vi "Diagonal Vents.vi"() -> ()   [LabVIEW 2020]
uses:
  <vilib>/regexp/Match Regular Expression.xnode
panel:
  out "Array":i32[][](array[numeric])
  out "Count":i32
  in  "Input":string="599,531 -> 599,32\n435,904 -> 435,489\n768,714 -> 768,187\n845,552 -> 596,801\n167,680 -> 167,445\n45,887 -> 45,346\n780,295 -> 179,896\n310,539 -> 602,831\n535,556 -> 349,556\n797,180 -> 797,62\n771,406 -> 120,406\n383,296 -> 383,918\n689,815 -> 73,199\n658,642 -> 658,333\n931,104 -> 708,104\n406,278 -> 406,29\n315,532 -> 773,74\n439,953 -> 289,953\n555,162 -> 695,302\n444,522 -> 444,828\n460,844 -> 460,972\n838,18 -> 143,713\n335,785 -> 335,485\n757,886 -> 757,327\n266,205 -> 273,205\n934,42 -> 19,957\n671,622 -> 263,214\n739,781 -> 739,332\n848,507 -> 848,394\n577,58 -> 461,174\n49,905 -> 921,33\n627,455 -> 205,455\n106,523 -> 974,523\n707,335 -> 707,313\n65,214 -> 712,214\n610,267 -> 610,403\n47,699 -> 565,181\n288,833 -> 709,833\n452,59 -> 452,632\n629,209 -> 125,209\n535,232 -> 535,342\n542,942 -> 542,753\n618,905 -> 552,905\n598,314 -> 976,314\n350,824 -> 17,824\n753,570 -> 753,617\n544,302 -> 259,302\n628,271 -> 628,379\n856,265 -> 856,792\n77,317 -> 77,122\n905,420 -> 905,687\n812,512 -> 812,411\n844,486 -> 771,559\n798,778 -> 798,215\n571,160 -> 278,453\n242,352 -> 227,352\n958,118 -> 167,909\n201,915 -> 201,564\n163,583 -> 163,279\n23,111 -> 23,883\n248,281 -> 331,281\n381,768 -> 900,768\n78,988 -> 78,326\n914,659 -> 247,659\n532,531 -> 520,531\n65,309 -> 734,978\n170,923 -> 399,694\n740,496 -> 196,496\n832,452 -> 816,452\n675,463 -> 878,463\n659,852 -> 560,852\n143,655 -> 227,655\n334,795 -> 334,978\n217,913 -> 368,913\n675,33 -> 503,33\n42,981 -> 811,981\n458,162 -> 722,162\n92,613 -> 92,542\n393,584 -> 393,252\n276,256 -> 725,705\n752,442 -> 752,789\n63,281 -> 744,281\n596,845 -> 35,284\n594,534 -> 964,164\n337,380 -> 337,511\n158,142 -> 75,225\n606,47 -> 606,111\n987,30 -> 62,955\n192,196 -> 428,196\n449,672 -> 449,77\n804,151 -> 804,255\n783,581 -> 287,581\n860,891 -> 69,100\n966,187 -> 761,392\n400,742 -> 278,742\n661,656 -> 592,587\n787,415 -> 787,771\n866,228 -> 417,228\n915,385 -> 505,385\n715,620 -> 715,633\n615,31 -> 615,940\n691,885 -> 527,885\n426,705 -> 351,705\n258,215 -> 258,949\n480,449 -> 480,710\n788,710 -> 788,67\n850,90 -> 597,90\n398,379 -> 18,759\n248,107 -> 665,524\n901,933 -> 208,240\n433,424 -> 110,424\n214,447 -> 389,272\n468,330 -> 468,928\n950,759 -> 332,759\n447,541 -> 420,541\n659,138 -> 604,83\n821,264 -> 95,264\n914,132 -> 46,132\n821,604 -> 821,57\n805,734 -> 85,14\n806,274 -> 164,916\n205,780 -> 205,133\n798,472 -> 361,472\n817,57 -> 127,747\n172,119 -> 922,869\n118,167 -> 55,167\n56,548 -> 344,836\n117,108 -> 940,931\n530,46 -> 530,785\n528,507 -> 729,708\n11,986 -> 987,10\n979,932 -> 76,29\n863,250 -> 210,903\n879,215 -> 891,215\n592,219 -> 592,528\n211,760 -> 211,347\n21,842 -> 633,230\n110,356 -> 110,254\n925,606 -> 444,125\n757,566 -> 757,498\n702,622 -> 637,622\n51,379 -> 365,379\n273,906 -> 273,494\n170,795 -> 929,36\n159,56 -> 435,56\n724,953 -> 724,735\n536,748 -> 901,748\n937,148 -> 937,510\n963,507 -> 863,507\n840,290 -> 840,221\n864,154 -> 55,963\n977,487 -> 685,487\n863,617 -> 210,617\n862,308 -> 291,879\n286,477 -> 286,276\n550,805 -> 550,489\n964,508 -> 821,651\n475,290 -> 789,290\n25,882 -> 25,349\n570,374 -> 604,374\n354,442 -> 514,282\n457,700 -> 360,700\n548,889 -> 548,502\n11,393 -> 11,829\n60,714 -> 781,714\n943,953 -> 972,924\n757,386 -> 465,386\n230,463 -> 27,463\n815,385 -> 326,385\n32,630 -> 378,976\n298,853 -> 298,644\n532,146 -> 23,146\n958,685 -> 737,464\n853,847 -> 79,73\n815,590 -> 815,961\n49,87 -> 751,789\n55,513 -> 55,378\n163,907 -> 574,907\n355,168 -> 355,836\n453,742 -> 674,742\n273,458 -> 685,458\n981,961 -> 958,984\n120,59 -> 401,59\n735,964 -> 395,964\n277,377 -> 277,646\n633,694 -> 633,707\n224,376 -> 976,376\n201,790 -> 293,790\n950,952 -> 12,14\n389,48 -> 356,48\n337,424 -> 166,424\n591,915 -> 591,456\n205,162 -> 942,162\n404,421 -> 404,748\n319,983 -> 608,694\n94,677 -> 94,853\n873,388 -> 873,617\n858,82 -> 858,890\n64,503 -> 64,787\n372,224 -> 50,546\n531,241 -> 960,670\n47,33 -> 975,961\n853,52 -> 271,634\n668,437 -> 668,719\n162,290 -> 843,290\n421,299 -> 944,822\n103,983 -> 103,324\n290,71 -> 290,686\n209,38 -> 546,38\n740,878 -> 378,878\n741,795 -> 741,916\n27,431 -> 445,431\n795,289 -> 795,759\n345,772 -> 775,772\n977,480 -> 512,15\n49,863 -> 49,659\n223,590 -> 779,590\n503,771 -> 917,771\n499,289 -> 935,725\n246,459 -> 246,395\n860,257 -> 656,257\n425,87 -> 425,603\n355,378 -> 355,23\n462,286 -> 462,358\n181,571 -> 181,732\n17,649 -> 476,649\n394,321 -> 394,293\n812,660 -> 515,957\n21,150 -> 799,928\n437,593 -> 437,372\n125,495 -> 373,743\n482,404 -> 482,420\n283,580 -> 283,234\n667,966 -> 827,806\n959,961 -> 959,931\n461,845 -> 206,845\n299,888 -> 299,836\n680,828 -> 680,855\n958,977 -> 26,45\n847,419 -> 290,976\n892,920 -> 892,180\n487,945 -> 487,445\n329,570 -> 583,570\n110,940 -> 989,61\n475,351 -> 882,351\n953,229 -> 429,229\n119,125 -> 749,125\n834,103 -> 212,725\n978,412 -> 978,343\n916,310 -> 758,310\n825,761 -> 720,761\n353,954 -> 353,795\n422,464 -> 422,356\n662,964 -> 836,790\n242,873 -> 242,570\n742,972 -> 797,972\n698,364 -> 360,26\n258,633 -> 19,872\n406,649 -> 406,685\n386,710 -> 925,710\n347,657 -> 524,480\n812,905 -> 554,647\n420,505 -> 420,231\n908,693 -> 908,724\n130,772 -> 130,898\n560,23 -> 560,987\n941,831 -> 941,544\n817,940 -> 132,255\n515,280 -> 515,811\n544,102 -> 568,102\n115,612 -> 67,660\n743,762 -> 743,152\n246,14 -> 691,459\n766,492 -> 673,492\n467,179 -> 351,63\n655,779 -> 655,524\n314,171 -> 314,108\n414,64 -> 502,64\n564,239 -> 894,239\n984,974 -> 56,46\n201,963 -> 201,223\n238,194 -> 238,832\n30,652 -> 477,652\n818,735 -> 582,971\n225,566 -> 673,566\n172,865 -> 74,865\n264,101 -> 264,812\n487,916 -> 979,916\n879,30 -> 10,899\n797,657 -> 797,136\n750,642 -> 593,799\n550,244 -> 418,376\n158,816 -> 668,816\n505,648 -> 303,648\n411,688 -> 263,688\n544,35 -> 771,35\n545,846 -> 286,846\n284,760 -> 284,929\n835,401 -> 708,401\n533,591 -> 545,591\n866,757 -> 475,757\n202,62 -> 907,767\n456,655 -> 456,123\n367,714 -> 225,714\n359,679 -> 926,679\n623,853 -> 623,865\n170,120 -> 213,120\n481,741 -> 481,435\n928,73 -> 41,960\n551,282 -> 551,265\n988,986 -> 12,10\n351,172 -> 791,172\n49,65 -> 952,968\n725,617 -> 691,617\n509,159 -> 697,159\n83,985 -> 83,968\n206,617 -> 334,489\n880,682 -> 966,768\n60,896 -> 60,617\n501,686 -> 49,234\n801,708 -> 738,771\n548,883 -> 548,33\n753,162 -> 29,162\n102,478 -> 102,295\n115,656 -> 637,134\n924,970 -> 924,963\n191,340 -> 191,515\n764,481 -> 523,481\n97,619 -> 97,890\n228,183 -> 228,624\n171,867 -> 68,867\n797,685 -> 167,685\n510,955 -> 464,955\n930,955 -> 233,258\n934,572 -> 934,900\n217,822 -> 797,242\n868,939 -> 369,440\n861,811 -> 861,36\n346,617 -> 346,153\n754,526 -> 754,426\n482,724 -> 482,21\n328,984 -> 976,984\n933,895 -> 325,287\n965,973 -> 232,240\n502,707 -> 767,972\n353,680 -> 815,218\n311,210 -> 311,157\n156,944 -> 928,172\n615,395 -> 101,909\n107,500 -> 528,921\n375,42 -> 375,796\n13,292 -> 818,292\n613,144 -> 613,541\n340,677 -> 340,406\n631,655 -> 744,655\n22,242 -> 723,943\n705,596 -> 980,321\n316,955 -> 316,515\n760,279 -> 44,279\n391,328 -> 391,724\n917,476 -> 917,668\n66,907 -> 913,60\n597,260 -> 362,25\n568,584 -> 568,297\n375,506 -> 375,300\n988,31 -> 72,947\n425,342 -> 154,342\n196,395 -> 899,395\n904,17 -> 94,17\n546,159 -> 751,159\n284,557 -> 175,448\n69,201 -> 697,201\n130,421 -> 224,421\n646,462 -> 637,453\n187,638 -> 621,638\n832,212 -> 416,212\n614,582 -> 348,582\n677,404 -> 677,709\n178,122 -> 915,859\n81,849 -> 223,849\n717,18 -> 646,18\n723,666 -> 974,666\n703,234 -> 130,234\n317,107 -> 106,107\n207,397 -> 207,375\n688,465 -> 982,171\n749,201 -> 610,201\n280,313 -> 827,860\n773,873 -> 917,873\n337,908 -> 337,155\n541,427 -> 385,583\n611,314 -> 131,794\n966,909 -> 104,47\n785,556 -> 346,556\n914,645 -> 914,718\n683,941 -> 657,915\n919,665 -> 310,56\n743,978 -> 779,978\n953,925 -> 953,854\n899,347 -> 705,347\n46,597 -> 46,255\n332,364 -> 922,954\n38,987 -> 832,193\n77,585 -> 77,262\n155,61 -> 734,640\n953,136 -> 655,136\n939,730 -> 158,730\n903,458 -> 393,458\n50,227 -> 50,249\n536,814 -> 536,242\n906,694 -> 259,47\n317,237 -> 853,773\n828,55 -> 509,55\n40,664 -> 341,965\n414,820 -> 53,459\n244,344 -> 272,344\n191,606 -> 308,606\n329,409 -> 329,960\n166,863 -> 938,91\n655,396 -> 291,760\n634,666 -> 625,666\n360,622 -> 360,550\n568,473 -> 840,201\n534,162 -> 534,823\n583,563 -> 583,521\n124,447 -> 124,79\n207,559 -> 207,649\n688,238 -> 26,900\n173,33 -> 117,33\n665,800 -> 665,86\n121,515 -> 121,132\n32,472 -> 32,960\n513,28 -> 513,299\n881,612 -> 881,415\n72,71 -> 977,976\n169,821 -> 111,821\n603,756 -> 254,756\n182,129 -> 182,824\n746,670 -> 942,670\n143,15 -> 72,86\n108,134 -> 963,989\n860,388 -> 834,362\n252,811 -> 473,811\n575,306 -> 575,368\n686,471 -> 686,38\n673,59 -> 673,861\n461,949 -> 491,949\n915,373 -> 330,958\n933,699 -> 588,699\n254,798 -> 254,498\n329,865 -> 329,926\n569,243 -> 659,243\n762,808 -> 921,967\n722,460 -> 68,460\n136,470 -> 355,470\n133,919 -> 56,842\n87,868 -> 853,102\n622,102 -> 446,102\n798,494 -> 135,494\n281,858 -> 281,172\n141,172 -> 765,796\n794,194 -> 102,886\n539,983 -> 539,895\n841,755 -> 841,365\n695,429 -> 166,958\n965,933 -> 899,933\n603,699 -> 603,708\n598,635 -> 844,635\n288,190 -> 288,946\n559,383 -> 423,383\n795,332 -> 409,718\n600,645 -> 478,645\n831,24 -> 905,24\n13,817 -> 606,224\n828,878 -> 96,146\n32,197 -> 32,891\n84,832 -> 84,756\n404,281 -> 404,781\n394,441 -> 489,536\n845,876 -> 589,876\n833,114 -> 833,834\n979,130 -> 979,238\n907,189 -> 396,700\n448,740 -> 714,474\n145,837 -> 100,837\n982,983 -> 38,39\n962,506 -> 962,764\n773,922 -> 975,922\n892,666 -> 904,654\n754,201 -> 459,496\n108,829 -> 108,894\n122,381 -> 122,484\n683,301 -> 630,354\n47,103 -> 897,953\n549,880 -> 942,487\n944,15 -> 44,915\n713,456 -> 713,402\n83,865 -> 239,865\n814,585 -> 814,105\n980,439 -> 685,439"
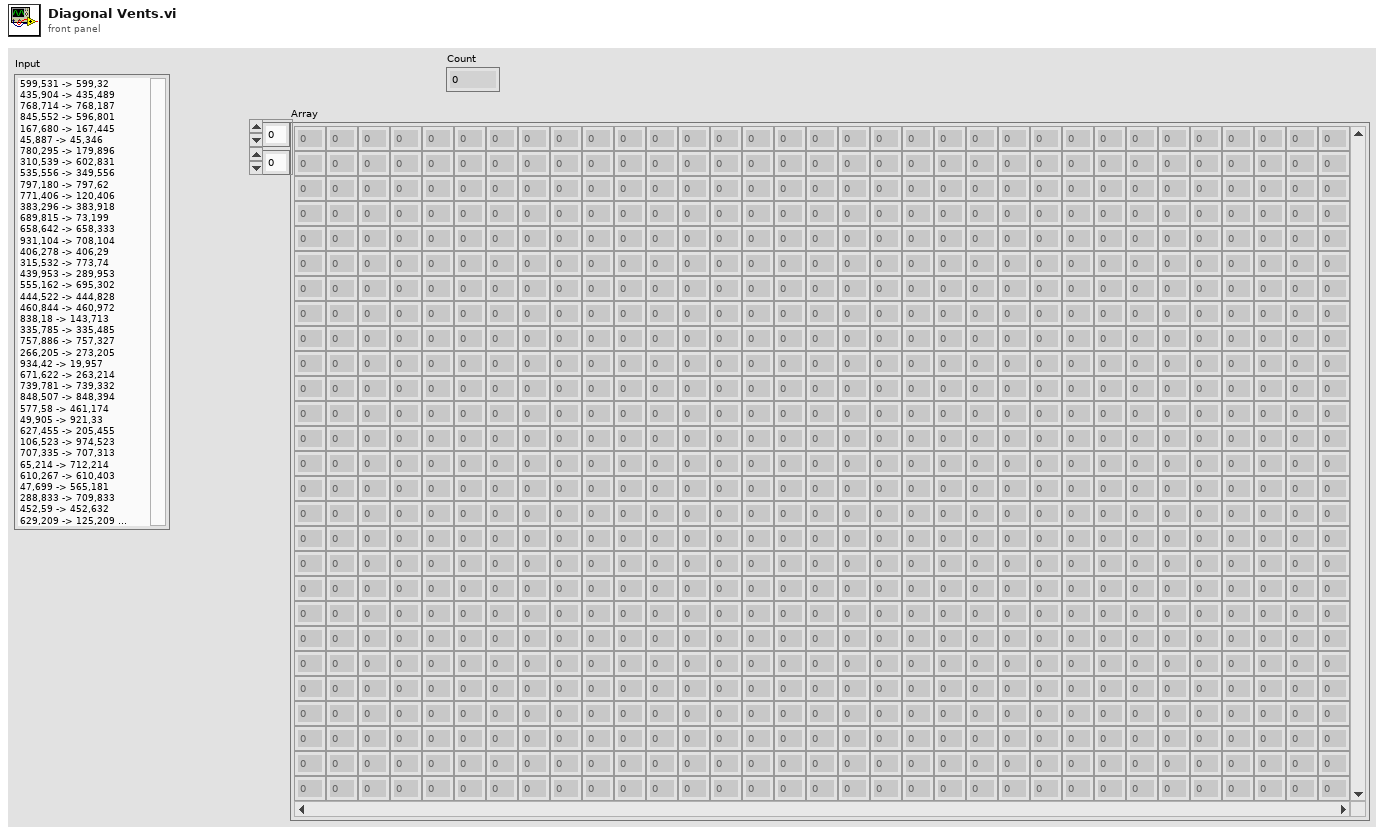
[diagram p1: front panel]
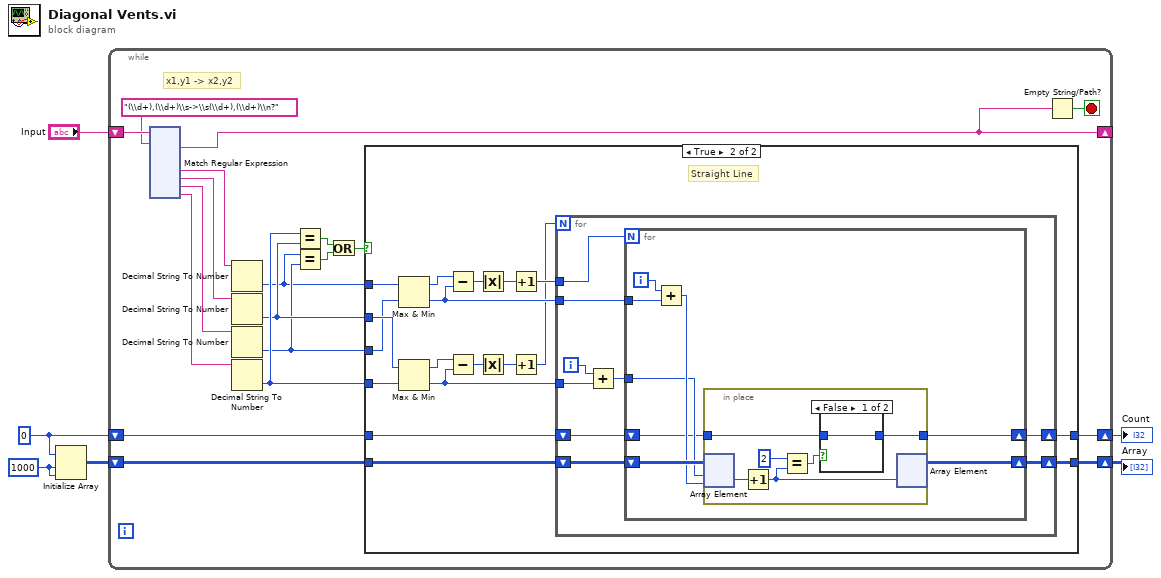
[diagram p0: block diagram]
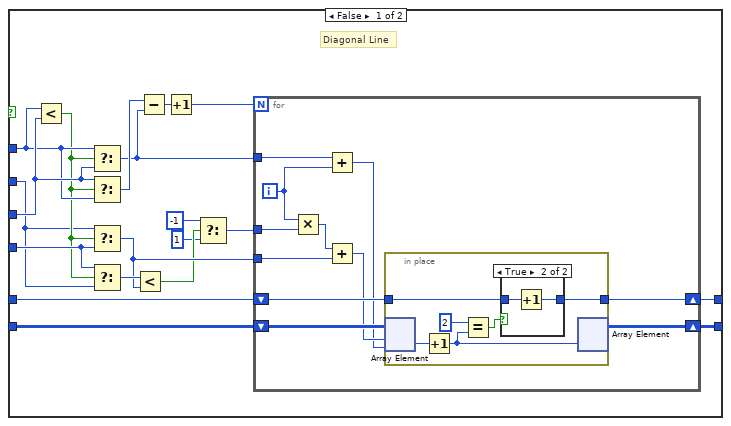
[diagram p2: hidden frame]
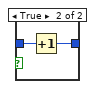
[diagram p4: hidden frame]
diagram:
  w3 = 0
  w6 = 1000 ("dimension size")
  n1 = Initialize Array(w3, w6, w6) -> (w4:i32[][])
  n2 = while {
    shift-right: [w19] -> _
    shift-left: "Input" -> [w25]
    shift-right: [w15] -> w1
    shift-left: w4 -> [w16]
    shift-right: [w14] -> w2
    shift-left: w3 -> [w17]
    stop <- w18 stop-if-true
    # "x1,y1 -> x2,y2"
    n3 = xnode "Match Regular Expression"("input string"=w25, "regular expression"="(\\d+),(\\d+)\\s->\\s(\\d+),(\\d+)\\n?") -> ("after match"=w19:string, "submatch 1"=w23:string, "submatch 2"=w22:string, "submatch 3"=w21:string, "submatch 4"=w20:string)  [unwired: 4 in, 4 out]
    n4 = Decimal String To Number(string=w23) -> (number=w7:i32)  [unwired: 2 in, 1 out]
    n5 = Decimal String To Number(string=w22) -> (number=w9:i32)  [unwired: 2 in, 1 out]
    n6 = Decimal String To Number(string=w21) -> (number=w8:i32)  [unwired: 2 in, 1 out]
    n7 = Decimal String To Number(string=w20) -> (number=w10:i32)  [unwired: 2 in, 1 out]
    n8 = Equal?(x=w10, y=w9) -> (x = y?=w13:bool)
    n9 = Equal?(x=w7, y=w8) -> (x = y?=w12:bool)
    n10 = Or(x=w13, y=w12) -> (x .or. y?=w11:bool)
    n11 = case shown="True" w11 {
      tunnel: w17 -> [w163 w201]
      tunnel: w16 -> [w162 w200]
      tunnel: [w160 w199] -> w15
      tunnel: [w161 w198] -> w14
      tunnel: w10 -> [w153 w191]
      tunnel: w9 -> [w151 w190]
      tunnel: w8 -> [w159 w189]
      tunnel: w7 -> [w158 w188]
      frame False {
        # "Diagonal Line"
        n12 = Less?(x=w158, y=w159) -> (x < y?=w152:bool)
        n13 = Select(t=w158, s=w152, f=w159) -> (s? t:f=w154:i32)
        n14 = Select(t=w159, s=w152, f=w158) -> (s? t:f=w157:i32)
        n15 = Select(t=w151, s=w152, f=w153) -> (s? t:f=w148:i32)
        n16 = Select(t=w153, s=w152, f=w151) -> (s? t:f=w150:i32)
        n17 = Less?(x=w150, y=w148) -> (x < y?=w147:bool)
        n18 = Subtract(x=w157, y=w154) -> (x-y=w156:i32)
        n19 = Increment(x=w156) -> (x+1=w155:i32)
        n20 = Select(t=-1, s=w147, f=1) -> (s? t:f=w149:i32)
        n21 = for {
          N: w155 -> [_]
          tunnel: w154 -> [w174]
          tunnel: w148 -> [w173]
          shift-right: [w168] -> w161
          shift-left: w163 -> [w171]
          shift-right: [w164] -> w160
          shift-left: w162 -> [w172]
          tunnel: w149 -> [w165]
          i -> [w166]
          n22 = Multiply(x=w166, y=w165) -> (x*y=w167:i32)
          n23 = Add(x=w174, y=w166) -> (x+y=w169:i32)
          n24 = Add(x=w167, y=w173) -> (x+y=w170:i32)
          n25 = in-place {
            in-place-border: w171 -> [w176]
            in-place-border: [w175] -> w168
            n26 = in-place-array #1(w172, w170, w169) -> (w180:i32)
            n27 = Increment(x=w180) -> (x+1=w179:i32)
            n28 = Equal?(x=2, y=w179) -> (x = y?=w177:bool)
            n29 = case shown="True" w177 {
              tunnel: w176 -> [w181 w183]
              tunnel: [w181 w182] -> w175
              frame False {
              }
              frame True {
                n30 = Increment(x=w183) -> (x+1=w182:i32)
              }
            }
            n31 = in-place-array #1(w179) -> (w164:i32[][])  [unwired: 2 out]
          }
        }
      }
      frame True {
        # "Straight Line"
        n32 = Max & Min(x=w188, y=w189) -> (max(x,y)=w197:i32, min(x,y)=w186:i32)
        n33 = Max & Min(x=w190, y=w191) -> (max(x,y)=w192:i32, min(x,y)=w185:i32)
        n34 = Subtract(x=w197, y=w186) -> (x-y=w196:i32)
        n35 = Subtract(x=w192, y=w185) -> (x-y=w193:i32)
        n36 = Absolute Value(x=w196) -> (abs(x)=w195:i32)
        n37 = Absolute Value(x=w193) -> (abs(x)=w194:i32)
        n38 = Increment(x=w195) -> (x+1=w187:i32)
        n39 = Increment(x=w194) -> (x+1=w184:i32)
        n40 = for {
          N: w184 -> [_]
          shift-right: [w204] -> w199
          shift-left: w200 -> [w206]
          tunnel: w185 -> [w209]
          tunnel: w186 -> [w210]
          shift-right: [w203] -> w198
          shift-left: w201 -> [w205]
          tunnel: w187 -> [w202]
          i -> [w208]
          n41 = Add(x=w208, y=w209) -> (x+y=w207:i32)
          n42 = for {
            N: w202 -> [_]
            tunnel: w210 -> [w218]
            tunnel: w207 -> [w214]
            shift-right: [w211] -> w204
            shift-left: w206 -> [w216]
            shift-right: [w212] -> w203
            shift-left: w205 -> [w213]
            i -> [w217]
            n43 = Add(x=w217, y=w218) -> (x+y=w215:i32)
            n44 = in-place {
              in-place-border: w213 -> [w220]
              in-place-border: [w219] -> w212
              n45 = in-place-array #2(w216, w214, w215) -> (w224:i32)
              n46 = Increment(x=w224) -> (x+1=w223:i32)
              n47 = Equal?(x=2, y=w223) -> (x = y?=w221:bool)
              n48 = case shown="False" w221 {
                tunnel: w220 -> [w225 w227]
                tunnel: [w225 w226] -> w219
                frame False {
                }
                frame True {
                  n49 = Increment(x=w227) -> (x+1=w226:i32)
                }
              }
              n50 = in-place-array #2(w223) -> (w211:i32[][])  [unwired: 2 out]
            }
          }
        }
      }
    }
    n51 = Empty String/Path?(string/path=w19) -> (empty?=w18:bool)
  }
  "Count" <- w2
  "Array" <- w1
